vi "RotateCount Value Change.vi"(10 "Rotate count":u32 caption="Maximum Number of Archived Files To Keep", 11 "References":T1) -> (0 "error out":errorcluster)   [LabVIEW 2015, in "TDMS datalogger editor node.lvclass"]
uses:
  TDMS datalogger editor node.lvclass
  <vilib>/NI/DCAF/Tag Editor Core/Table API/Table Manager/object ref.ctl
  <vilib>/NI/DCAF/Tag Editor Core/Configuration Editor/Classes/Engine Parent/Engine Parent Editor Node.lvclass
  <vilib>/NI/DCAF/Tag Editor Core/Configuration Editor/Classes/Module editor node/module editor node.lvclass
  TDMS datalogger editor node.lvclass/TDMS datalogger editor node.ctl
  module/configuration/TDMS datalogger configuration.lvclass/TDMS datalogger configuration.ctl
  module/configuration/Read logrotate_options.vi
  module/configuration/Write logrotate_options.vi
  module/configuration/TDMS datalogger configuration.lvclass
  <vilib>/NI/DCAF/Tag Editor Core/Table API/Table Manager/Table Manager.lvclass
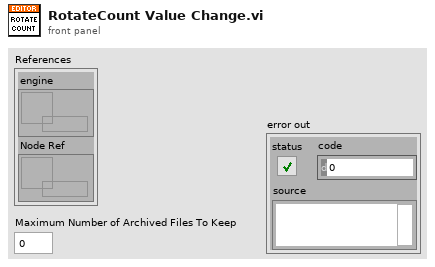
[diagram p1: front panel]
types:
  T1 = typedef "Table Manager.lvlib/Table Manager.lvclass/object ref.ctl" = cluster{"engine":refnum<data-value>, "Node Ref":refnum<data-value>}
  T2 = typedef "LogRotate.lvclass/options.ctl" = cluster{"max file size (bytes)":i64, "rotate count":u32, "max age (days)":dbl, "No archive dir":bool, "Archive dir":path}
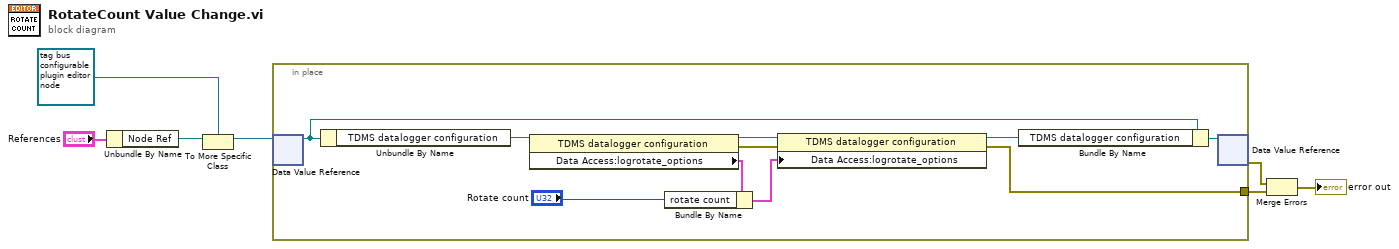
[diagram p0: block diagram]
diagram:
  n1 = Unbundle By Name("References") -> ("Node Ref"=w6:refnum<data-value>)
  n2 = To More Specific Class(target class=refnum<data-value> refnum ("data value reference"), reference=w6) -> (specific class reference=w4:refnum<data-value>)  [unwired: 1 in, 1 out]
  n3 = in-place {
    in-place-border: [w9] -> w3
    n4 = in-place-dvr #1(w4) -> (w12:refnum<class "TDMS datalogger editor node.lvclass">)  [unwired: 1 out]
    n5 = Unbundle By Name(w12) -> ("TDMS datalogger configuration"=w17:refnum<class "TDMS datalogger configuration.lvclass">)
    n6 = property class="TDMS datalogger configuration"(reference=w17) -> (reference out=w15:refnum<class "TDMS datalogger configuration.lvclass">, error out=w14:errorcluster, "Data Access:logrotate_options"=w16:T2)  [unwired: 1 in]
    n7 = Bundle By Name(cluster=w16, "rotate count"="Rotate count") -> (w13:T2)
    n8 = property class="TDMS datalogger configuration"(reference=w15, error in=w14, "Data Access:logrotate_options"=w13) -> (reference out=w11:refnum<class "TDMS datalogger configuration.lvclass">, error out=w9:errorcluster)
    n9 = Bundle By Name(cluster=w12, "TDMS datalogger configuration"=w11) -> (w10:refnum<class "TDMS datalogger editor node.lvclass">)
    n10 = in-place-dvr #1(w10) -> (w1:errorcluster)  [unwired: 1 out]
  }
  n11 = Merge Errors(w1, w3) -> (→"error out":errorcluster)
